vi "Exercício_2_Arduíno_Correto.vi"() -> ()   [LabVIEW 2017]
uses:
  <vilib>/LabVIEW Interface for Arduino/Type Defs/Board Type.ctl
  <vilib>/LabVIEW Interface for Arduino/Type Defs/Connection Type.ctl
  <vilib>/LabVIEW Interface for Arduino/Type Defs/Pin Mode.ctl
  <vilib>/LabVIEW Interface for Arduino/LabVIEW Interface for Arduino.lvlib
panel:
  out "Peças Altas":bool
  in  "Sensor 3":bool
  out "Peça não uniforme":bool
  out "Peça Baixa":bool
  in  "Sensor 2":bool
  in  "B LIGA":bool
  in  "Sensor 1":bool
  out "ESTEIRA ON":bool
  in  "stop":bool
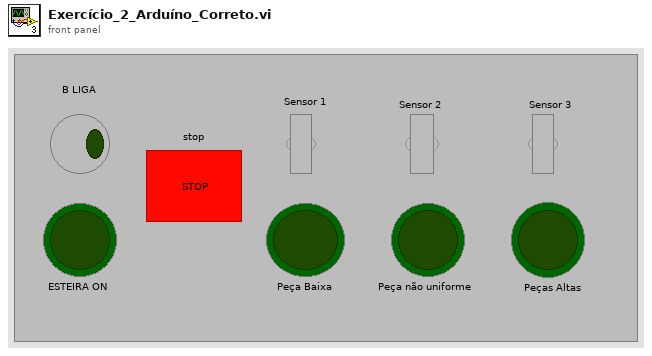
[diagram p1: front panel]
types:
  T1 = typedef "LabVIEW Interface for Arduino.lvlib/Pin Mode.ctl" = enum8{"Input", "Output"}
  T2 = typedef "LabVIEW Interface for Arduino.lvlib/Connection Type.ctl" = enum8{"USB / Serial", "XBEE", "BlueSmirf (Bluetooth)"}
  T3 = typedef "LabVIEW Interface for Arduino.lvlib/Board Type.ctl" = enum16{"Uno", "Dimuelanove w/Atmega 328", "Mega 2560"}
  T4 = typedef "LabVIEW Interface for Arduino.lvlib/Arduino Resource.ctl" = cluster{"VISA resource":refnum<visa-resource-name>, "Board Type":T3, "Connection Type":enum8{"USB / Serial"}, "Bytes Per Packet (15)":u8}
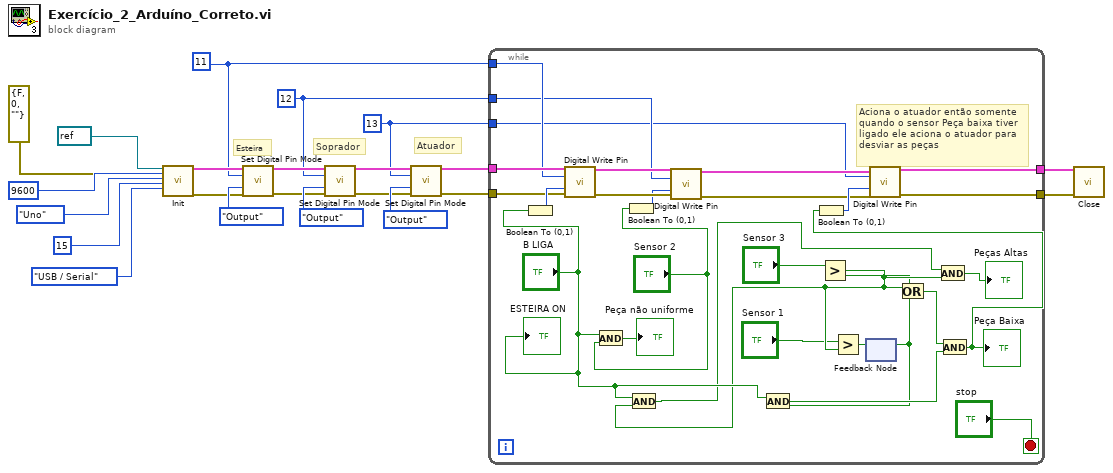
[diagram p0: block diagram]
diagram:
  w1 = u8 13 ("Digital I/O Pin")
  w4 = u8 12 ("Digital I/O Pin")
  w5 = u8 11 ("Digital I/O Pin")
  # "Atuador"
  # "Soprador"
  # "Esteira"
  n1 = call <vilib>:"Init.vi"("VISA resource"=refnum<visa-resource-name> refnum, "Baud Rate (115200)"=u32 9600, "Board Type (Uno)"=Board_Type."Uno", "Bytes Per Packet (15)"=u32 15, "Connection Type (USB/Serial)"=Connection_Type."USB / Serial", "error in"=errorcluster {"status"=FALSE, "code"=0, "source"=""}) -> ("Arduino Resource"=w7:T4, "error out"=w6:errorcluster)  [unwired: 12 in]
  n2 = call <vilib>:"Set Digital Pin Mode.vi"("Arduino Resource"=w7, "Digital I/O Pin"=w5, "Pin Mode (Input)"=Pin_Mode."Output", "error in"=w6) -> ("Arduino Resource"=w14:T4, "error out"=w13:errorcluster)  [unwired: 10 in]
  n3 = call <vilib>:"Set Digital Pin Mode.vi"("Arduino Resource"=w14, "Digital I/O Pin"=w4, "Pin Mode (Input)"=Pin_Mode."Output", "error in"=w13) -> ("Arduino Resource"=w11:T4, "error out"=w10:errorcluster)  [unwired: 10 in]
  n4 = call <vilib>:"Set Digital Pin Mode.vi"("Arduino Resource"=w11, "Digital I/O Pin"=w1, "Pin Mode (Input)"=Pin_Mode."Output", "error in"=w10) -> ("Arduino Resource"=w9:T4, "error out"=w8:errorcluster)  [unwired: 10 in]
  n5 = while {
    tunnel: w9 -> [w48]
    tunnel: w8 -> [w47]
    tunnel: w5 -> [w46]
    tunnel: w4 -> [w43]
    tunnel: [w38] -> w3
    tunnel: [w37] -> w2
    tunnel: w1 -> [w36]
    stop <- "stop" stop-if-true
    # "Aciona o atuador então somente quando o sensor Peça baixa tiver ligado ele aciona o atuador para desviar as peças"
    n6 = Boolean To (0,1)(Boolean="B LIGA") -> (0, 1=w50:i16)
    n7 = call <vilib>:"Digital Write Pin.vi"("Arduino Resource"=w48, "Digital I/O Pin (0)"=w46, "Value (0)"=w50, "error in"=w47) -> ("Arduino Resource"=w45:T4, "error out"=w44:errorcluster)  [unwired: 10 in]
    n8 = And(x="B LIGA", y="Sensor 2") -> (x .and. y?=→"Peça não uniforme":bool)
    n9 = Boolean To (0,1)(Boolean="Sensor 2") -> (0, 1=w42:i16)
    n10 = call <vilib>:"Digital Write Pin.vi"("Arduino Resource"=w45, "Digital I/O Pin (0)"=w43, "Value (0)"=w42, "error in"=w44) -> ("Arduino Resource"=w39:T4, "error out"=w40:errorcluster)  [unwired: 10 in]
    n11 = feedback #1() -> (w23:bool)  [unwired: 1 in]
    n12 = And(x="B LIGA", y=w23) -> (x .and. y?=w32:bool)
    n13 = Greater?(x="Sensor 3", y=w23) -> (0:w26:bool)
    n14 = And(x="B LIGA", y=w26) -> (x .and. y?=w28:bool)
    n15 = Greater?(x="Sensor 1", y=w26) -> (0:w24:bool)
    n16 = feedback-in #1(w24) -> ()
    n17 = Or(x=w26, y=w23) -> (x .or. y?=w31:bool)
    n18 = And(x=w28, y=w26) -> (x .and. y?=→"Peças Altas":bool)
    n19 = And(x=w31, y=w32) -> (x .and. y?=w30:bool)
    "Peça Baixa" <- w30
    n20 = Boolean To (0,1)(Boolean=w30) -> (0, 1=w41:i16)
    n21 = call <vilib>:"Digital Write Pin.vi"("Arduino Resource"=w39, "Digital I/O Pin (0)"=w36, "Value (0)"=w41, "error in"=w40) -> ("Arduino Resource"=w38:T4, "error out"=w37:errorcluster)  [unwired: 10 in]
    "ESTEIRA ON" <- "B LIGA"
  }
  n22 = call <vilib>:"Close.vi"("Arduino Resource"=w3, "error in"=w2) -> ()  [unwired: 13 in, 1 out]
